vi "RT Driver VI.vi"(6 "Device Clock":string, 9 "Device Inputs FIFO":refnum<k33>, 10 "Device Outputs FIFO":refnum<k33>, 11 "Device Reference":T1 format="%.0x") -> ()   [LabVIEW 2015, in "Host Heartbeat Engine.lvlib"]
uses:
  Host Heartbeat Engine.lvlib
  <vilib>/NI Veristand/Custom Device API/Custom Device Item Ref.ctl
  Shared/Constants.vi
  <vilib>/NI Veristand/Custom Device API/Get Item Property (U16).vi
  <vilib>/NI Veristand/Custom Device Tools/Custom Device Utility Library/Custom Device Utility Library.lvlib
  Shared/Host Heartbeat Shared.lvlib
  <vilib>/NI Veristand/Custom Device API/Custom Device API.lvlib
panel:
  in  "Initialization Status Notifier":refnum<notifier>
  in  "Status Notifier":refnum<notifier>
  # "Custom Device Template\nv1.0"
  # "Use this template as a starting point for creating a custom device code module. The input controls shown here are specially named controls that the system will use to provide the device loop with data. The controls are not required for the device loop to run. For instance, if the device doesn't produce any output data, then you don't need the Device Outputs FIFO control. If you do use these controls, however, they need to have these exact names to be functional."
  # "The optional status notifier element is used to notify the RT engine of the last state of the custom device, and to indicate the device has completed execution. If this control is not used, a default No Error value is returned to the system when the device finishes execution.\n\nNote: This error state is not checked until the system shuts down. Use an output status channel to send more immediate status values to the system."
  # "This optional input can be used to send the VeriStand Engine the final status of the custom device initalization process. If this control exists on the custom device front panel, the VeriStand Engine will wait for a status update before starting up. If the custom device reports an error, that will abort the execution of the current configuration in the VeriStand Engine.\n\nThis control can be deleted if the custom device does not need to send the initialization status update."
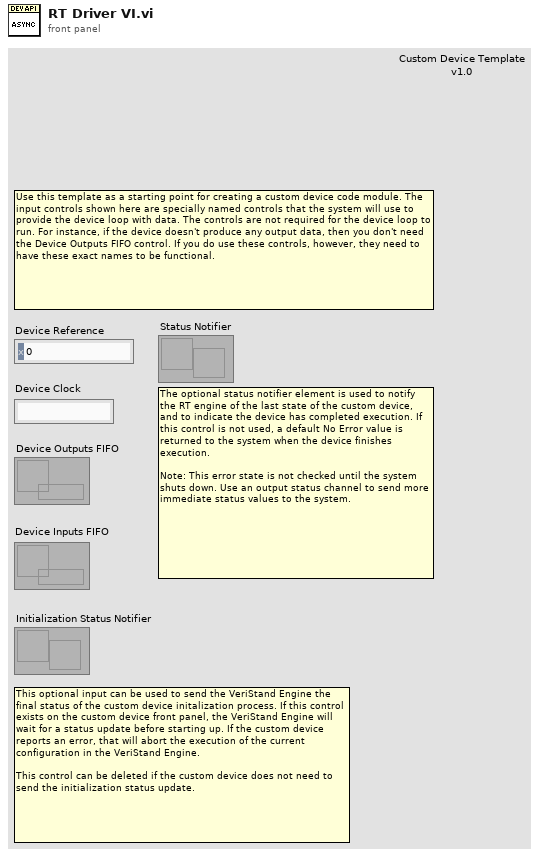
[diagram p1: front panel]
types:
  T1 = typedef "Custom Device API.lvlib/Custom Device Item Ref.ctl" = u64
  T2 = enum16{"Standard", "Buffered", "CRLF", "Immediate"}
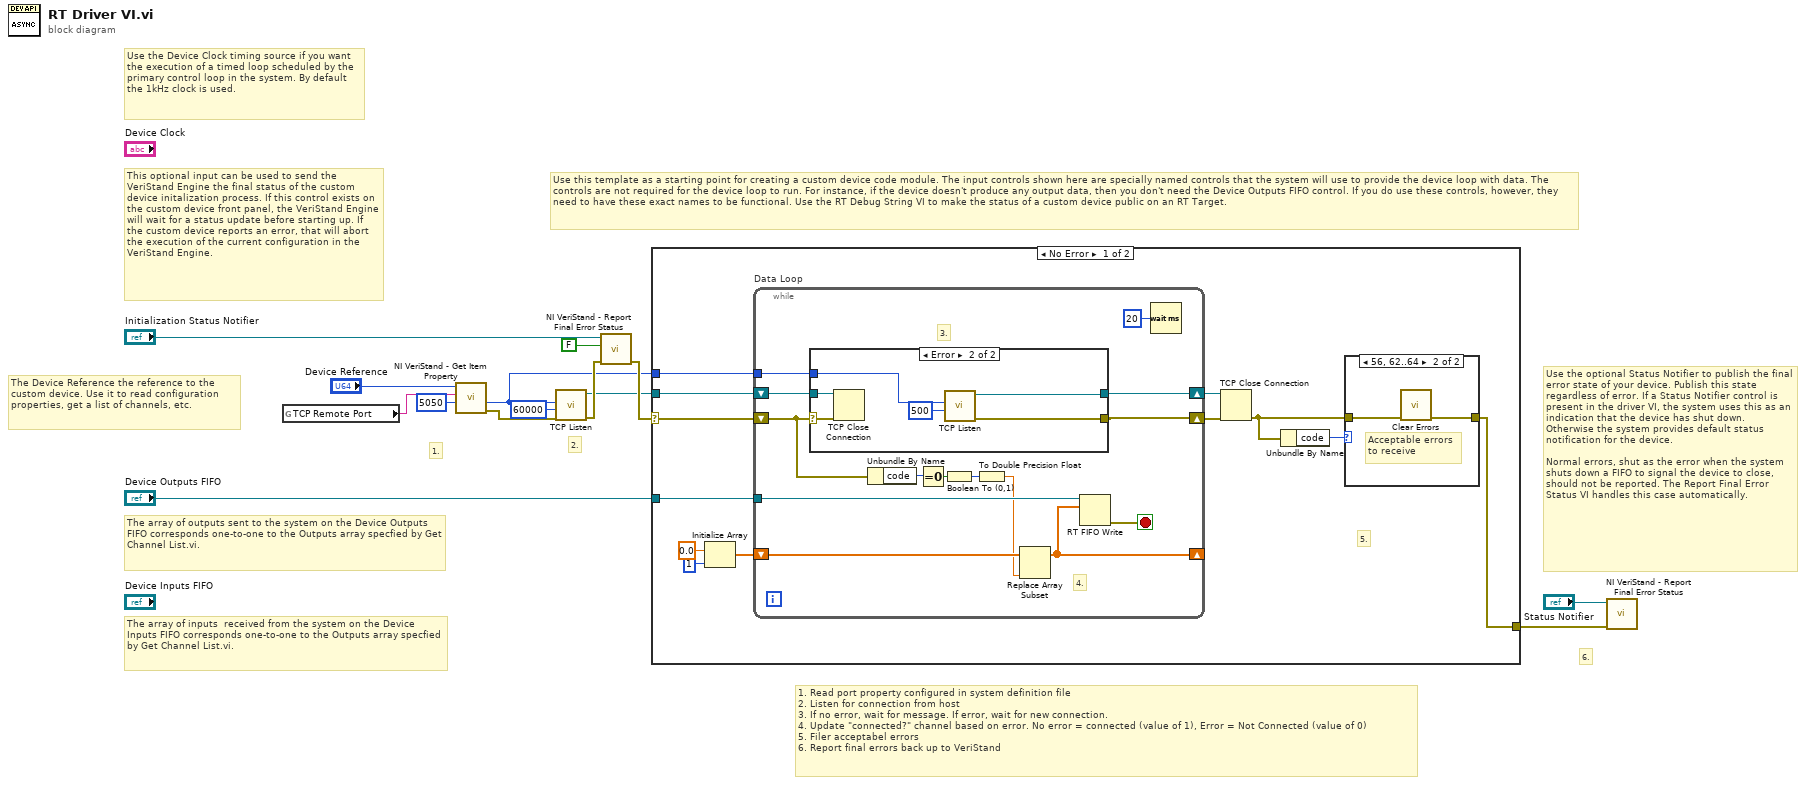
[diagram p0: block diagram]
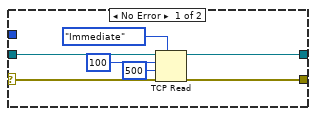
[diagram p3: hidden frame]
diagram:
  # "1. Read port property configured in system definition file\n2. Listen for connection from host\n3. If no error, wait for message. If error, wait for new connection.\n4. Update \"connected?\" channel based on error. No error = connected (value of 1), Error = Not Connected (value of 0)\n5. Filer acceptabel errors\n6. Report final errors back up to VeriStand"
  # "6."
  # "2."
  # "1."
  # "This optional input can be used to send the VeriStand Engine the final status of the custom device initalization process. If this control exists on the custom device front panel, the VeriStand Engine will wait for a status update before starting up. If the custom device reports an error, that will abort the execution of the current configuration in the VeriStand Engine."
  # "The array of inputs  received from the system on the Device Inputs FIFO corresponds one-to-one to the Outputs array specfied by Get Channel List.vi."
  # "Use the optional Status Notifier to publish the final error state of your device. Publish this state regardless of error. If a Status Notifier control is present in the driver VI, the system uses this as an indication that the device has shut down. Otherwise the system provides default status notification for the device.\n\nNormal errors, shut as the error when the system shuts down a FIFO to signal the device to close, should not be reported. The Report Final Error Status VI handles this case automatically."
  # "The array of outputs sent to the system on the Device Outputs FIFO corresponds one-to-one to the Outputs array specfied by Get Channel List.vi."
  # "The Device Reference the reference to the custom device. Use it to read configuration properties, get a list of channels, etc."
  # "Use the Device Clock timing source if you want the execution of a timed loop scheduled by the primary control loop in the system. By default the 1kHz clock is used."
  # "Use this template as a starting point for creating a custom device code module. The input controls shown here are specially named controls that the system will use to provide the device loop with data. The controls are not required for the device loop to run. For instance, if the device doesn't produce any output data, then you don't need the Device Outputs FIFO control. If you do use these controls, however, they need to have these exact names to be functional. Use the RT Debug String VI to make the status of a custom device public on an RT Target."
  n1 = global read "Constants.vi" "TCP Remote Port"() -> (w4:string)
  n2 = call-poly <vilib>:"NI VeriStand - Get Item Property.vi"("Default Value"=u16 5050, "Property Name"=w4, "Item Ref in"="Device Reference") -> ("error out"=w2:errorcluster, "Value"=w1:u16)  [unwired: 5 in, 2 out]
  n3 = call <vilib>:"TCP Listen.vi"("error in (no error)"=w2, "timeout ms (wait forever: -1)"=60000, "port"=w1) -> ("error out"=w8:errorcluster, "connection ID"=w6:refnum<k5>)  [unwired: 4 in, 3 out]
  n4 = call <vilib>:"NI VeriStand - Report Final Error Status.vi"("error in (no error)"=w8, "Filter FIFO & Shutdown Errors (T)"=FALSE ("Filter FIFO Errors (T)"), "Status Notifier"="Initialization Status Notifier") -> ("error out"=w7:errorcluster)  [unwired: 8 out]
  n5 = case shown="No Error" w7 {
    selector: w7 -> [w19 w57]
    tunnel: "Device Outputs FIFO" -> [w26 _]
    tunnel: [w16 w57] -> w11
    tunnel: w6 -> [w20 _]
    tunnel: w1 -> [w15 _]
    frame No Error {
      # "5."
      n6 = Initialize Array(0.0 ("element"), 1 ("dimension size")) -> (w23:dbl[])
      n7 = while "Data Loop" {
        shift-right: [w33] -> w21
        shift-left: w19 -> [w32]
        tunnel: w26 -> [w43]
        shift-right: [w38] -> _
        shift-left: w23 -> [w40]
        shift-right: [w34] -> w22
        shift-left: w20 -> [w35]
        tunnel: w15 -> [w30]
        stop <- w36 stop-if-true
        # "4."
        # "3."
        n8 = case shown="Error" w32 {
          selector: w32 -> [w48 w56]
          tunnel: w35 -> [w50 w55]
          tunnel: [w49 w53] -> w33
          tunnel: [w47 w52] -> w34
          tunnel: w30 -> [_ w51]
          frame No Error {
            n9 = TCP Read(connection ID=w50, bytes to read=100, error in (no error)=w48, 7:T2."Immediate" ("mode (standard)"), 9:500 ("timeout ms (25000)")) -> (connection ID out=w47:refnum<k5>, error out=w49:errorcluster)  [unwired: 1 out]
          }
          frame Error {
            n10 = TCP Close Connection(connection ID=w55, error in (no error)=w56) -> ()  [unwired: 1 in, 2 out]
            n11 = call <vilib>:"TCP Listen.vi"("timeout ms (wait forever: -1)"=500, "port"=w51) -> ("error out"=w53:errorcluster, "connection ID"=w52:refnum<k5>)  [unwired: 5 in, 3 out]
          }
        }
        n12 = Unbundle By Name(w32) -> ("code"=w42:i32)
        n13 = Equal To 0?(x=w42) -> (x = 0?=w41:bool)
        n14 = Boolean To (0,1)(Boolean=w41) -> (0, 1=w39:i16)
        n15 = To Double Precision Float(number=w39) -> (double precision float=w37:dbl)
        n16 = Replace Array Subset(array=w40, new element=w37) -> (w38:dbl[])  [unwired: 1 in]
        n17 = RT FIFO Write(0:w43, 1:w38) -> (11:w36:errorcluster)  [unwired: 2 in, 4 out]
        n18 = Wait (ms)(milliseconds to wait=u32 20) -> ()  [unwired: 1 out]
      }
      n19 = TCP Close Connection(connection ID=w22, error in (no error)=w21) -> (error out=w17:errorcluster)  [unwired: 1 in, 1 out]
      n20 = Unbundle By Name(w17) -> ("code"=w18:i32)
      n21 = case shown="56, 62..64" w18 {
        tunnel: w17 -> [w27 w29]
        tunnel: [w27 w28] -> w16
        frame 0, Default {
        }
        frame 56, 62..64 {
          # "Acceptable errors\nto receive"
          n22 = call <vilib>:"Clear Errors.vi"("error in (no error)"=w29) -> ("error out"=w28:errorcluster)  [unwired: 5 in, 1 out]
        }
      }
    }
    frame Error {
    }
  }
  n23 = call <vilib>:"NI VeriStand - Report Final Error Status.vi"("error in (no error)"=w11, "Status Notifier"="Status Notifier") -> ()  [unwired: 1 in, 9 out]
